vi "CalibrationWithRamp.vi"() -> ()   [LabVIEW 2009]
uses:
  <vilib>/DAQmx/write.llb/DAQmx Write (Analog 1D DBL NChan 1Samp).vi
  DAQ Read Actions.ctl
  CalibrationRampState.ctl
panel:
  in  "Ramp Voltage":dbl[](array[numeric])
  out "Control Voltage":dbl[](array[numeric])
  in  "rate":dbl=100.0
  in  "samples per channel":i32=30
  out "Servo Error Reading":dbl[](array[numeric])
  in  "Command Voltage Task":refnum<k21>="Command Channels"
  in  "Readings Task":refnum<k21>="All Readings"
  in  "Write error in (no error)":errorcluster
  out "Read error out":errorcluster
  out "Write error out":errorcluster
  in  "Read error in (no error)":errorcluster
  out "Load Cell \nReading":dbl[](array[numeric])
  out "LVDT Reading":dbl[](array[numeric])
  in  "Command Voltage Input":T2 {"Actuator Z2" min=-10.0 max=10.0 step=0.1 scale=-10.0..10.0; "Actuator Z3" min=-10.0 max=10.0 step=0.1 scale=-10.0..10.0; "Actuator X2" min=-10.0 max=10.0 step=0.1 scale=-10.0..10.0; "Actuator Y1" min=-10.0 max=10.0 step=0.1 scale=-10.0..10.0; "Actuator Z1" min=-10.0 max=10.0 step=0.1 scale=-10.0..10.0; "Actuator X1" min=-10.0 max=10.0 step=0.1 scale=-10.0..10.0}
  in  "Quit":bool
  # "LBCB CALIBRATION PROGRAM"
  # "Channel Order:\nX1 X2 Y1 Z1 Z2 Z3"
  # "Channel Order:\nX1 X2 Y1 Z1 Z2 Z3\n\nLVDT Readings\nLoadcell Readings\nServo Errors"
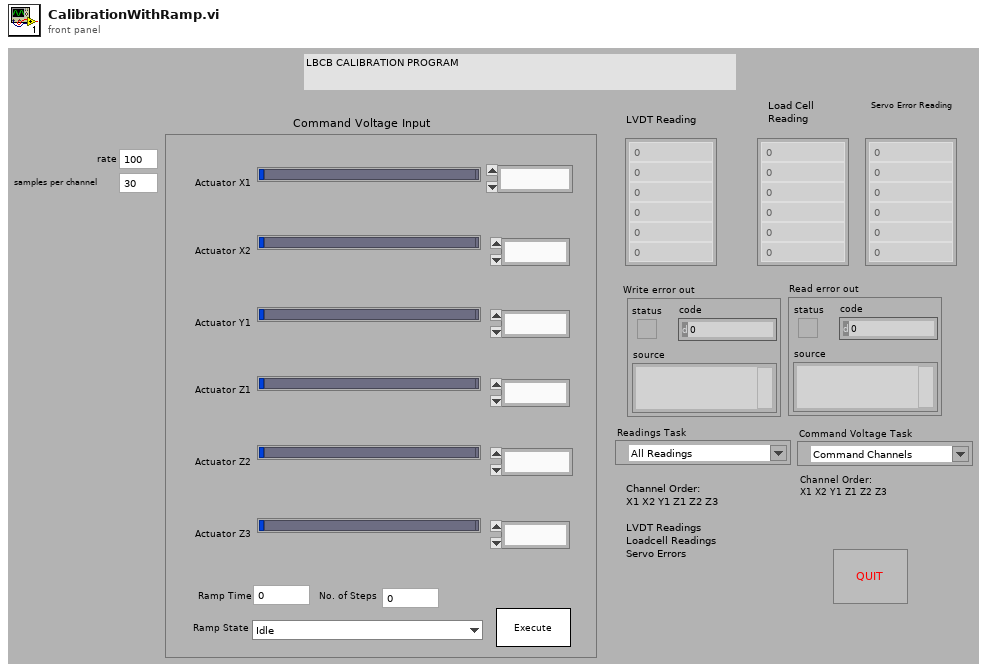
[diagram p1: front panel]
types:
  T1 = typedef "CalibrationRampState.ctl" = enum16{"Idle", "Start Ramp", "Ramping"}
  T2 = cluster{"Actuator X1":dbl, "Actuator Z1":dbl, "Actuator Y1":dbl, "Actuator X2":dbl, "Actuator Z3":dbl, "Actuator Z2":dbl, "Execute":bool, "Ramp State":T1, "Ramp Time":dbl, "No. of Steps":dbl}
  T3 = typedef "DAQ Read Actions.ctl" = enum16{"Start", "Read", "Stop"}
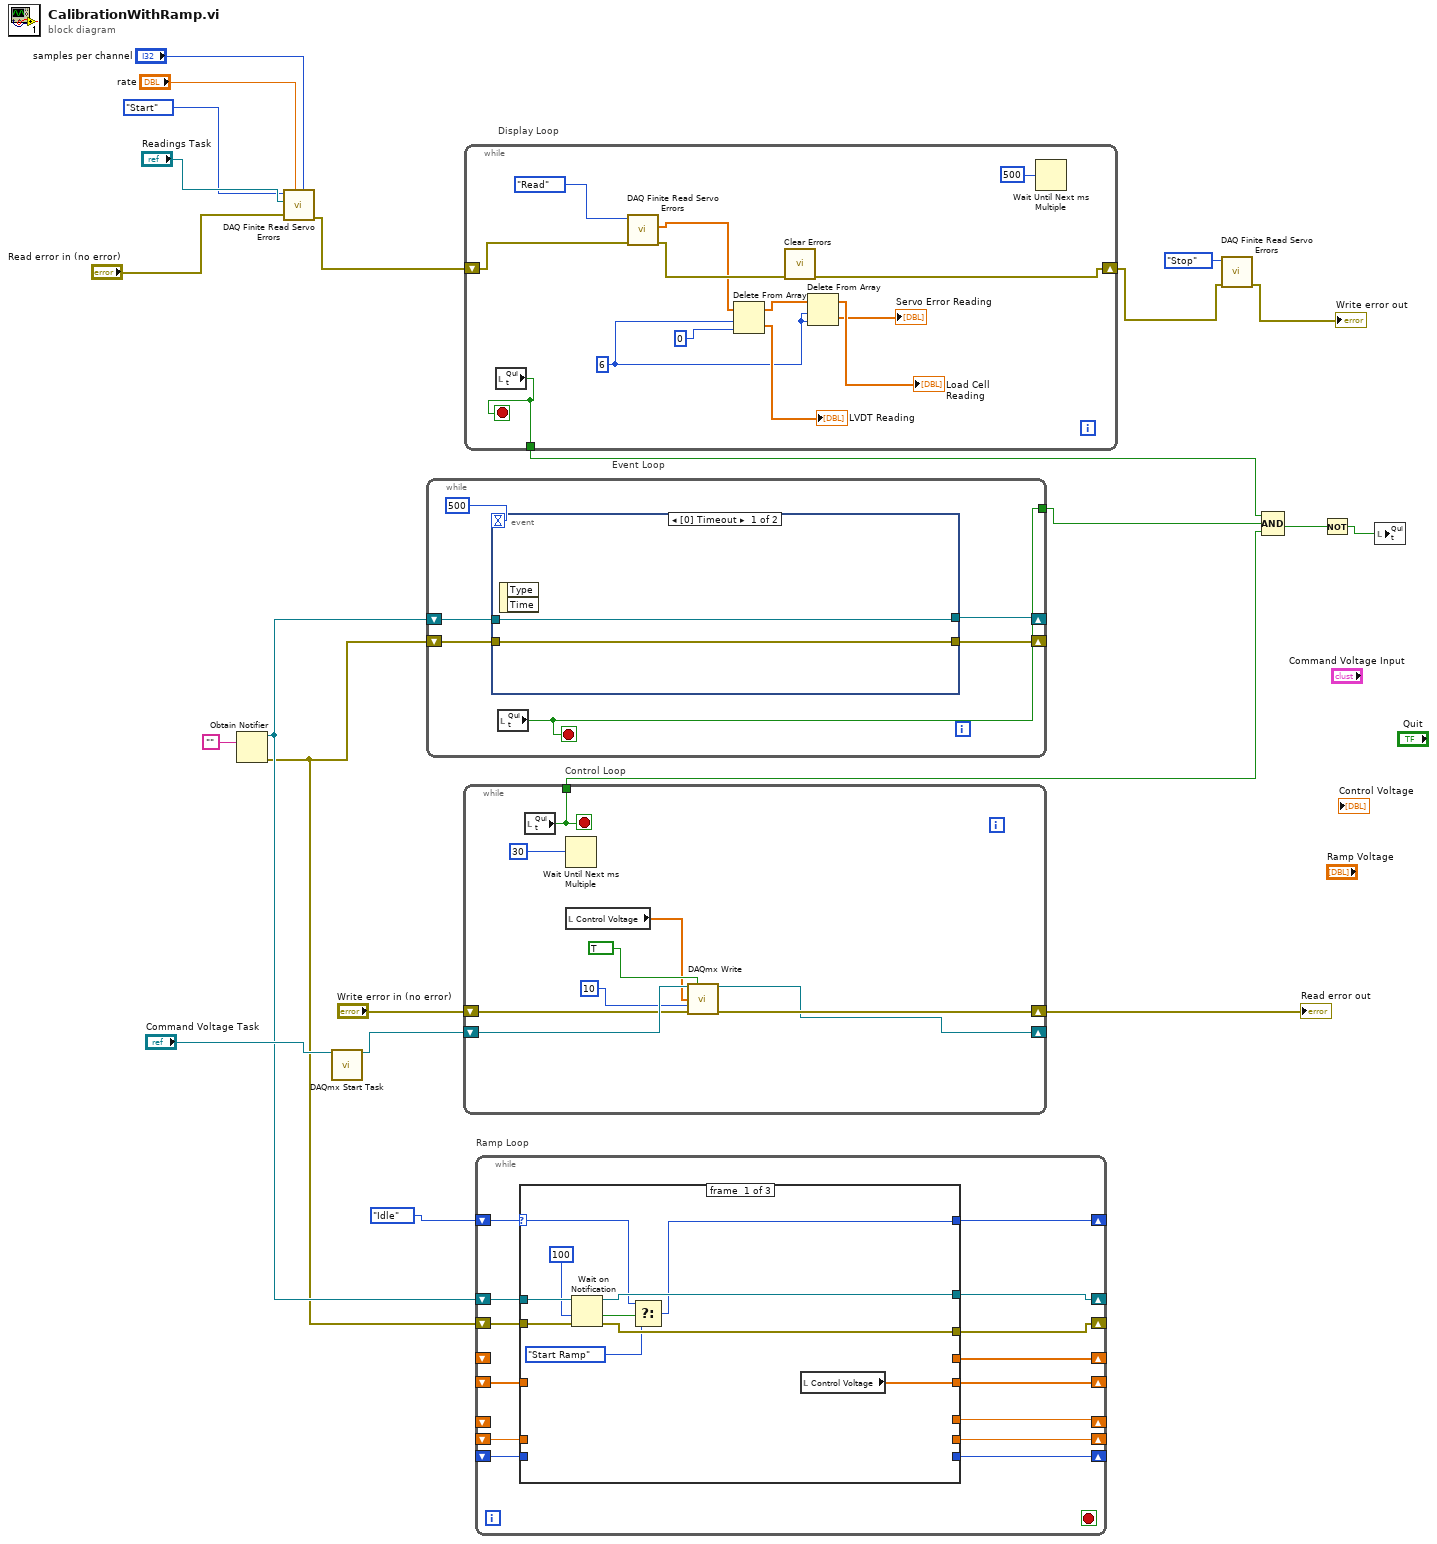
[diagram p0: block diagram]
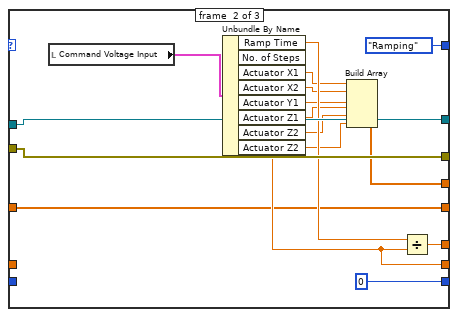
[diagram p2: hidden frame]
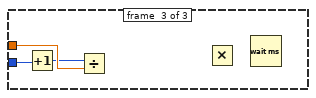
[diagram p3: hidden frame]
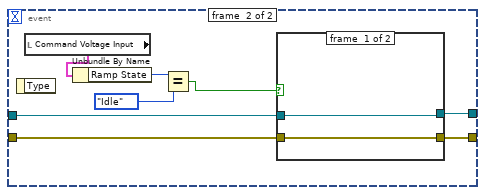
[diagram p4: hidden frame]
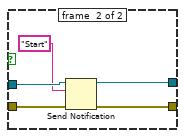
[diagram p5: hidden frame]
diagram:
  n1 = Obtain Notifier(notification data type="") -> (notifier out=w2:refnum<notifier>, error out=w1:errorcluster)  [unwired: 3 in, 1 out]
  n2 = call "DAQ Finite Read Servo Errors.vi"("samples per channel"="samples per channel", "rate"="rate", "error in"="Read error in (no error)", "task/channels in"="Readings Task", "Action"=DAQ_Read_Actions."Start") -> ("error out"=w10:errorcluster)  [unwired: 6 out]
  n3 = call <vilib>:"DAQmx Start Task.vi"("task/channels in"="Command Voltage Task") -> ("task out"=w22:refnum<k21>)  [unwired: 1 in, 13 out]
  n4 = while "Event Loop" {
    tunnel: [w27] -> w18
    shift-right: [w23] -> _
    shift-left: w1 -> [w25]
    shift-right: [w24] -> _
    shift-left: w2 -> [w26]
    stop <- w27 stop-if-true
    n5 = event shown="[0] Timeout" {
      selector: _ -> [_ _]
      dyn-events: _ -> [_ _]
      timeout: 500 -> [_ _]
      tunnel: w26 -> [w30 w34]
      tunnel: w25 -> [w29 w33]
      tunnel: [w30 w32] -> w24
      tunnel: [w29 w31] -> w23
      event #0 {
        n6 = event-data() -> ()  [unwired: 3 out]
      }
      event #1 {
        n7 = event-data() -> ()  [unwired: 2 out]
        n8 = local read "Command Voltage Input"() -> (w38:T2)
        n9 = Unbundle By Name(w38) -> ("Ramp State"=w37:T1)
        n10 = Equal?(x=w37, y=enum16{"Idle", "Start Ramp", "Ramping"}."Idle") -> (x = y?=w35:bool)
        n11 = case shown="False" w35 {
          tunnel: w34 -> [w40 w45]
          tunnel: w33 -> [w39 w43]
          tunnel: [w40 w42] -> w32
          tunnel: [w39 w41] -> w31
          frame #0 {
          }
          frame #1 {
            n12 = Send Notification(notification="Start", notifier=w45, error in (no error)=w43) -> (notifier out=w42:refnum<notifier>, error out=w41:errorcluster)
          }
        }
      }
    }
    n13 = local read "Quit"() -> (w27:bool)
  }
  n14 = while "Control Loop" {
    shift-right: [w51] -> _
    shift-left: w22 -> [w54]
    shift-right: [w52] -> w20
    shift-left: "Write error in (no error)" -> [w53]
    tunnel: [w47] -> w14
    stop <- w47 stop-if-true
    n15 = local read "Quit"() -> (w47:bool)
    n16 = Wait Until Next ms Multiple(millisecond multiple=30) -> ()  [unwired: 1 out]
    n17 = local read "Control Voltage"() -> (w46:dbl[])
    n18 = call-poly <vilib>:"DAQmx Write.vi"("task/channels in"=w54, "auto start"=TRUE, "data"=w46, "timeout"=10, "error in"=w53) -> ("task out"=w51:refnum<k21>, "error out"=w52:errorcluster)  [unwired: 9 out]
  }
  "Read error out" <- w20
  n19 = while "Display Loop" {
    shift-right: [w64] -> w7
    shift-left: w10 -> [w58]
    tunnel: [w66] -> w16
    stop <- w66 stop-if-true
    w62 = 6
    n20 = local read "Quit"() -> (w66:bool)
    n21 = call "DAQ Finite Read Servo Errors.vi"("error in"=w58, "Action"=DAQ_Read_Actions."Read") -> ("error out"=w57:errorcluster, "Average"=w56:dbl[])  [unwired: 3 in, 5 out]
    n22 = Delete From Array(array=w56, length=w62, index=0) -> (deleted portion=→"LVDT Reading":dbl[], array with subset deleted=w63:dbl[])
    n23 = call <vilib>:"Clear Errors.vi"("error in (no error)"=w57) -> ("error out"=w64:errorcluster)  [unwired: 6 out]
    n24 = Delete From Array(array=w63, length=w62, index=w62) -> (deleted portion=→"Servo Error Reading":dbl[], array with subset deleted=→"Load Cell \nReading":dbl[])
    n25 = Wait Until Next ms Multiple(millisecond multiple=500) -> ()  [unwired: 1 out]
  }
  n26 = while "Ramp Loop" {
    shift-right: [w76] -> _
    shift-left: CalibrationRampState."Idle" ("Ramp State") -> [w81]
    shift-right: [w78] -> _
    shift-left: w2 -> [w80]
    shift-right: [w77] -> _
    shift-left: w1 -> [w79]
    shift-right: [w75] -> _
    shift-left: _ -> [_]
    shift-right: [w73] -> _
    shift-left: _ -> [w68]
    shift-right: [w74] -> _
    shift-left: _ -> [w69]
    shift-right: [w72] -> _
    shift-left: _ -> [w70]
    shift-right: [w71] -> _
    shift-left: _ -> [_]
    stop <- _ stop-if-true
    n27 = case shown="\"Ramping\"" w81 {
      selector: w81 -> [w85 _ _]
      tunnel: w80 -> [w91 w106 _]
      tunnel: w79 -> [w90 w107 _]
      tunnel: [w87 w106 _] -> w78
      tunnel: [w86 w107 _] -> w77
      tunnel: [w84 CalibrationRampState."Ramping" ("f") _] -> w76
      tunnel: [_ w102 _] -> w75
      tunnel: [_ 0 _] -> w74
      tunnel: [_ w100 _] -> w73
      tunnel: [w82 w92 _] -> w72
      tunnel: [_ w93 _] -> w71
      tunnel: w70 -> [_ w92 _]
      tunnel: w69 -> [_ _ w110]
      tunnel: w68 -> [_ _ w109]
      frame #0 {
        n28 = Wait on Notification(notifier=w91, timeout in ms (-1)=100, error in (no error)=w90) -> (notifier out=w87:refnum<notifier>, timed out?=w88:bool, error out=w86:errorcluster)  [unwired: 1 in, 1 out]
        n29 = Select(t=w85, s=w88, f=CalibrationRampState."Start Ramp") -> (s? t:f=w84:T1)
        n30 = local read "Control Voltage"() -> (w82:dbl[])
      }
      frame #1 {
        n31 = local read "Command Voltage Input"() -> (w104:T2)
        n32 = Unbundle By Name(w104) -> ("Ramp Time"=w103:dbl, "No. of Steps"=w100:dbl, "Actuator X1"=w99:dbl, "Actuator X2"=w98:dbl, "Actuator Y1"=w97:dbl, "Actuator Z1"=w96:dbl, "Actuator Z2"=w95:dbl, "Actuator Z2"=w94:dbl)
        n33 = Build Array(w99, w98, w97, w96, w95, w94) -> (w93:dbl[])
        n34 = Divide(x=w103, y=w100) -> (x/y=w102:dbl)
      }
      frame #2 {
        n35 = Increment(x=w110) -> (x+1=w108:i32)
        n36 = Divide(x=w108, y=w109) -> ()  [unwired: 1 out]
        n37 = Multiply() -> ()  [unwired: 2 in, 1 out]
        n38 = Wait (ms)() -> ()  [unwired: 1 in, 1 out]
      }
    }
  }
  n39 = call "DAQ Finite Read Servo Errors.vi"("error in"=w7, "Action"=DAQ_Read_Actions."Stop") -> ("error out"=→"Write error out":errorcluster)  [unwired: 3 in, 6 out]
  n40 = Compound Arithmetic op=AND(w16, w18, w14) -> (w17:bool)
  n41 = Not(x=w17) -> (.not. x?=w15:bool)
  n42 = local write "Quit"(w15) -> ()
